vi "BRig_dataExp_LED_baseline_l2.vi"() -> (2 "output_LED_baseline_l2":i32)   [LabVIEW 2014]
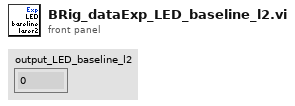
[diagram p1: front panel]
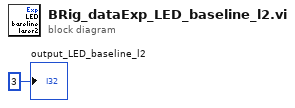
[diagram p0: block diagram]
diagram:
  "output_LED_baseline_l2" <- 3 ("output_iBlock")
